vi "GetVISAResourceName.vi"(0 "object in":refnum<class "Valve.lvclass">, 5 "error in (no error)":errorcluster) -> (14 "object out":refnum<class "Valve.lvclass">, 15 "VISA resource name":refnum<visa-resource-name>, 19 "error out":errorcluster)   [LabVIEW 2019, in "Valve.lvclass"]
uses:
  Valve.lvclass
  Valve.lvclass/Valve.ctl
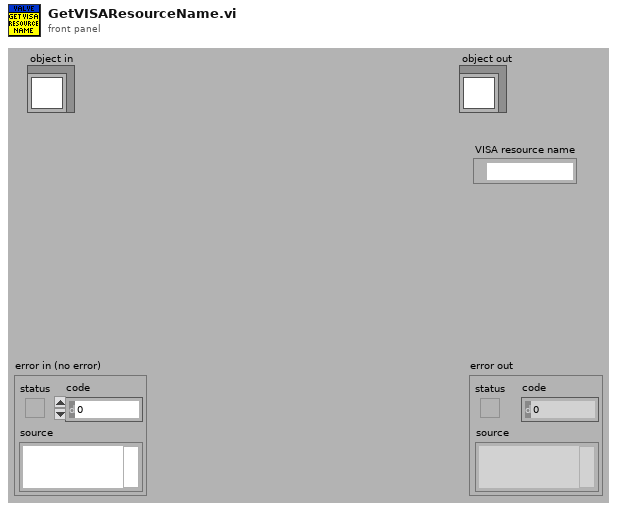
[diagram p1: front panel]
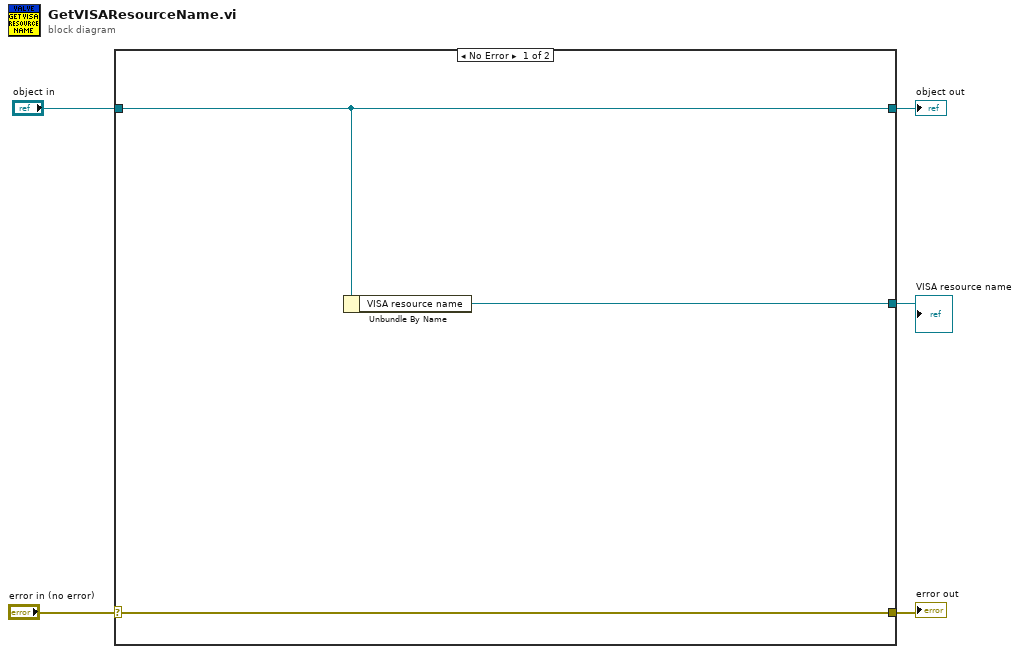
[diagram p0: block diagram]
diagram:
  n1 = case shown="No Error" "error in (no error)" {
    selector: "error in (no error)" -> [w7 w10]
    tunnel: [w7 w10] -> w4
    tunnel: [w6 w9] -> w2
    tunnel: "object in" -> [w6 w9]
    tunnel: [w8 _] -> w1
    frame No Error {
      n2 = Unbundle By Name(w6) -> ("VISA resource name"=w8:refnum<visa-resource-name>)
    }
    frame Error {
    }
  }
  "error out" <- w4
  "object out" <- w2
  "VISA resource name" <- w1
